vi "PSTR-Options Dialog.vi"(0 "Cluster In":T2={"Sample rate (Hz)"=20000.0, "Nfft"=0, "save raw"=FALSE, "sep"=0.0, "Window"=enum."NONE"}) -> (4 "Cluster out":T2={"Sample rate (Hz)"=20000.0, "Nfft"=0, "save raw"=FALSE, "sep"=0.0, "Window"=enum."NONE"}, 8 "Canceled?":bool)   [LabVIEW 2020]
uses:
  Typedefs/PSTR-Hidden Params.ctl
  Typedefs/PSTR-Window Shape.ctl
  epl-vi-lib/Utility VIs/Buttons/KCheckmarkBoolean 2.ctl
panel:
  in  "Window":enum16{"NONE", "Hamming"}(ring)
  in  "Save raw data":T1
  in  "Nfft":i32 caption="FFT length"
  in  "Sampling rate (Hz)":dbl
  in  "Cancel":bool
  in  "OK":bool
  # "Options"
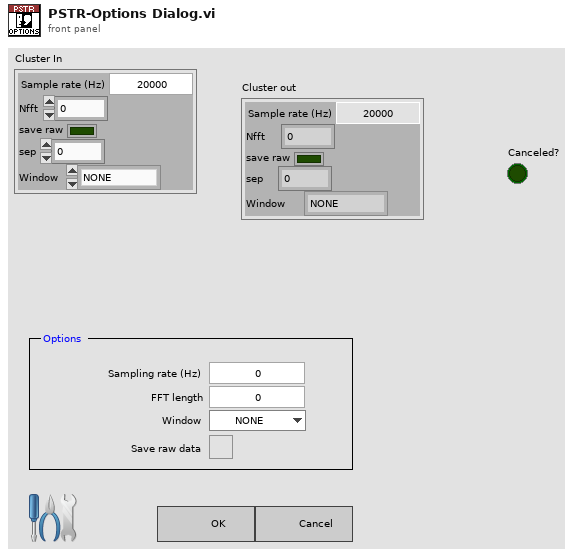
[diagram p1: front panel]
types:
  T1 = typedef "KCheckmarkBoolean 2.ctl" = bool
  T2 = typedef "PSTR-Hidden Params.ctl" = cluster{"Sample rate (Hz)":dbl, "Nfft":i32, "save raw":bool, "sep":dbl, "Window":T3}
  T3 = typedef "PSTR-Window Shape.ctl" = enum16{"NONE", "Hamming"}
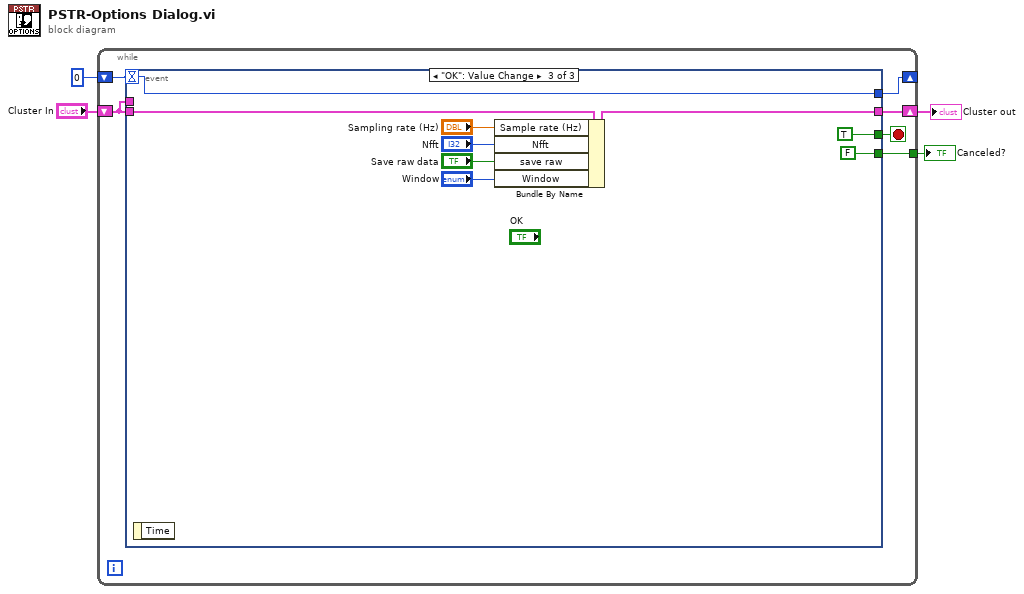
[diagram p0: block diagram]
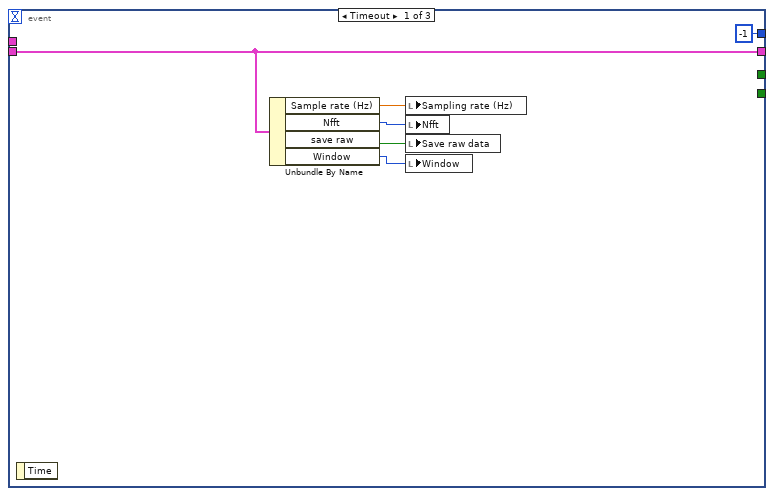
[diagram p2: hidden frame]
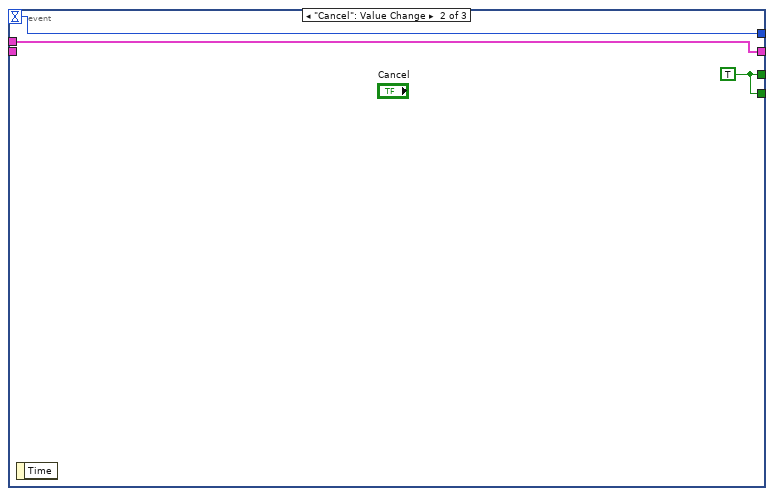
[diagram p3: hidden frame]
diagram:
  n1 = while {
    shift-right: [w9] -> _
    shift-left: 0 -> [w10]
    tunnel: [w6] -> w1
    shift-right: [w8] -> w2
    shift-left: "Cluster In" -> [w5]
    stop <- w7 stop-if-true
    n2 = event shown="[2] \"OK\": Value Change" {
      selector: _ -> [_ _ _]
      dyn-events: _ -> [_ _ _]
      timeout: w10 -> [_ w19 w27]
      tunnel: [-1 w19 w27] -> w9
      tunnel: w5 -> [w15 _ w28]
      tunnel: [w15 w17 w24] -> w8
      tunnel: [_ w18 TRUE] -> w7
      tunnel: [_ w18 FALSE] -> w6
      tunnel: w5 -> [_ w17 _]
      event Timeout {
        n3 = event-data() -> ()  [unwired: 1 in, 1 out]
        n4 = Unbundle By Name(w15) -> ("Sample rate (Hz)"=w14:dbl, "Nfft"=w13:i32, "save raw"=w12:bool, "Window"=w11:T3)
        n5 = local write "Sampling rate (Hz)"(w14) -> ()
        n6 = local write "Nfft"(w13) -> ()
        n7 = local write "Save raw data"(w12) -> ()
        n8 = local write "Window"(w11) -> ()
      }
      event "Cancel": Value Change {
        w18 = TRUE
        n9 = event-data() -> ()  [unwired: 1 in, 1 out]
      }
      event "OK": Value Change {
        n10 = event-data() -> ()  [unwired: 1 in, 1 out]
        n11 = Bundle By Name(cluster=w28, "Sample rate (Hz)"="Sampling rate (Hz)", "Nfft"="Nfft", "save raw"="Save raw data", "Window"="Window") -> (w24:T2)
      }
    }
  }
  "Cluster out" <- w2
  "Canceled?" <- w1
